vi "realTimeDisplay_AS3.vi"() -> ()   [LabVIEW 2016]
uses:
  <userlib>/RSA_API/RSA_API.lvlib
panel:
  in  "Cluster":T1 {"verticalUnit" items=["SpectrumVerticalUnit_dBm", "SpectrumVerticalUnit_Watt", "SpectrumVerticalUnit_Volt", "SpectrumVerticalUnit_Amp", "SpectrumVerticalUnit_dBmV"]; "window" items=["SpectrumWindow_Kaiser", "SpectrumWindow_Mil6dB", "SpectrumWindow_BlackmanHarris", "SpectrumWindow_Rectangle", "SpectrumWindow_FlatTop", "SpectrumWindow_Hann"]}
  out "settings out 2":T2 {"window" items=["SpectrumWindow_Kaiser", "SpectrumWindow_Mil6dB", "SpectrumWindow_BlackmanHarris", "SpectrumWindow_Rectangle", "SpectrumWindow_FlatTop", "SpectrumWindow_Hann"]; "verticalUnit" items=["SpectrumVerticalUnit_dBm", "SpectrumVerticalUnit_Watt", "SpectrumVerticalUnit_Volt", "SpectrumVerticalUnit_Amp", "SpectrumVerticalUnit_dBmV"]}
  in  "Done":bool
  in  "center freq":dbl
  in  "refLevel in":dbl
  in  "Trace number":u32(ring) items=["SpectrumTrace1", "SpectrumTrace2", "SpectrumTrace3"]
  out "traceData out":sgl[](graph)
  out "outTracePoints out":i32
  out "Trace Ready":bool
  out "enable out":bool
  out "refLevel out":dbl
  out "cf out":dbl
  in  "deviceID":i32
  out "deviceType out":string
  out "deviceSerial out":string
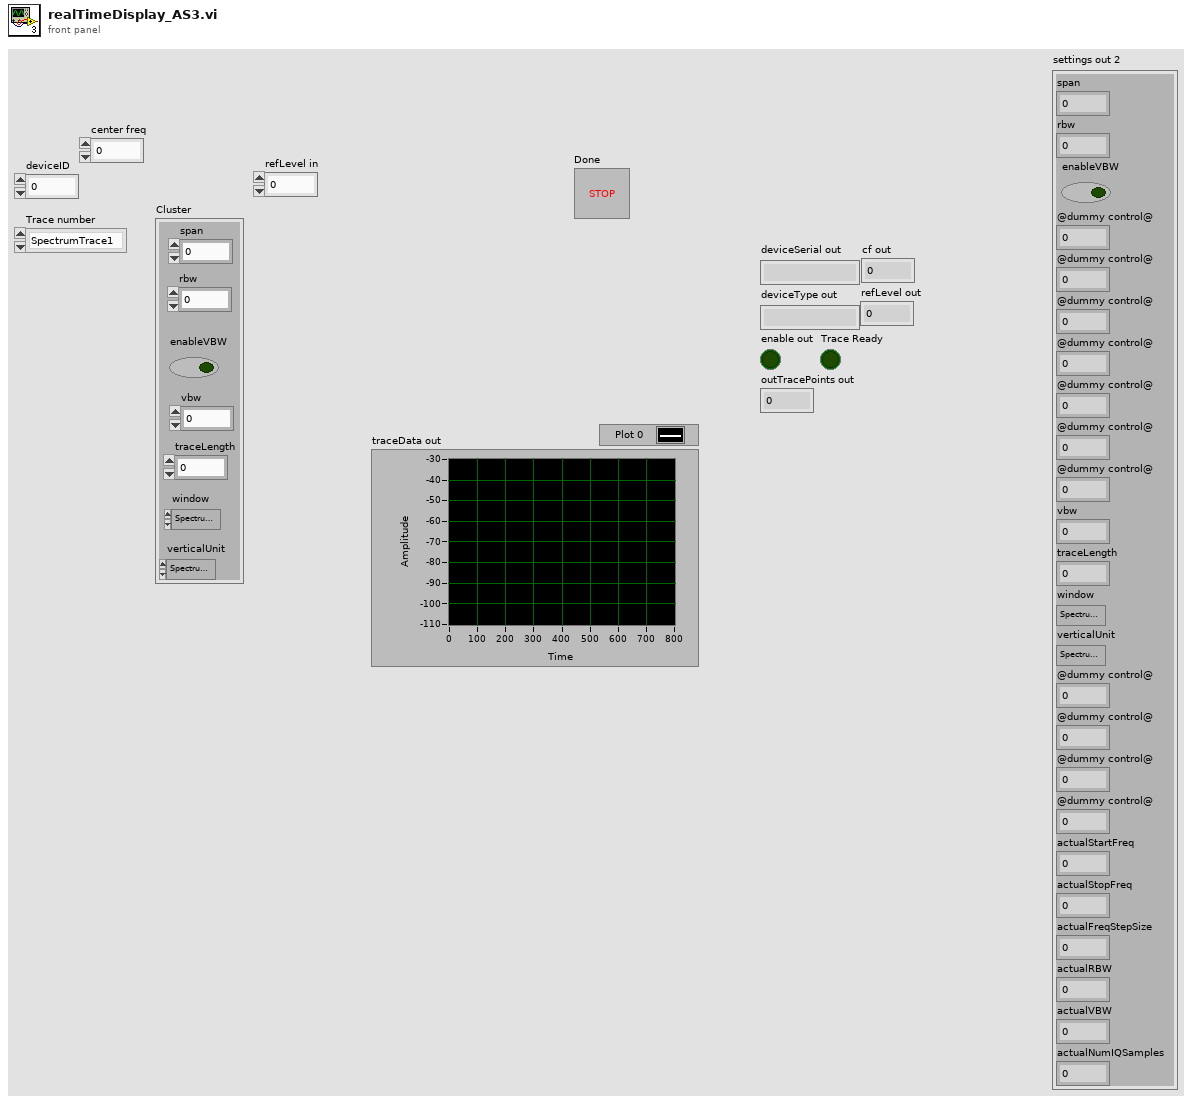
[diagram p1: front panel]
types:
  T1 = cluster{"span":dbl, "rbw":dbl, "enableVBW":bool, "vbw":dbl, "traceLength":i32, "window":u32, "verticalUnit":u32}
  T2 = cluster{"span":dbl, "rbw":dbl, "enableVBW":bool, "@dummy control@":i8, "@dummy control@":i8, "@dummy control@":i8, "@dummy control@":i8, "@dummy control@":i8, "@dummy control@":i8, "@dummy control@":i8, "vbw":dbl, "traceLength":i32, "window":u32, "verticalUnit":u32, "@dummy control@":i8, "@dummy control@":i8, "@dummy control@":i8, "@dummy control@":i8, "actualStartFreq":dbl, "actualStopFreq":dbl, "actualFreqStepSize":dbl, "actualRBW":dbl, "actualVBW":dbl, "actualNumIQSamples":i32}
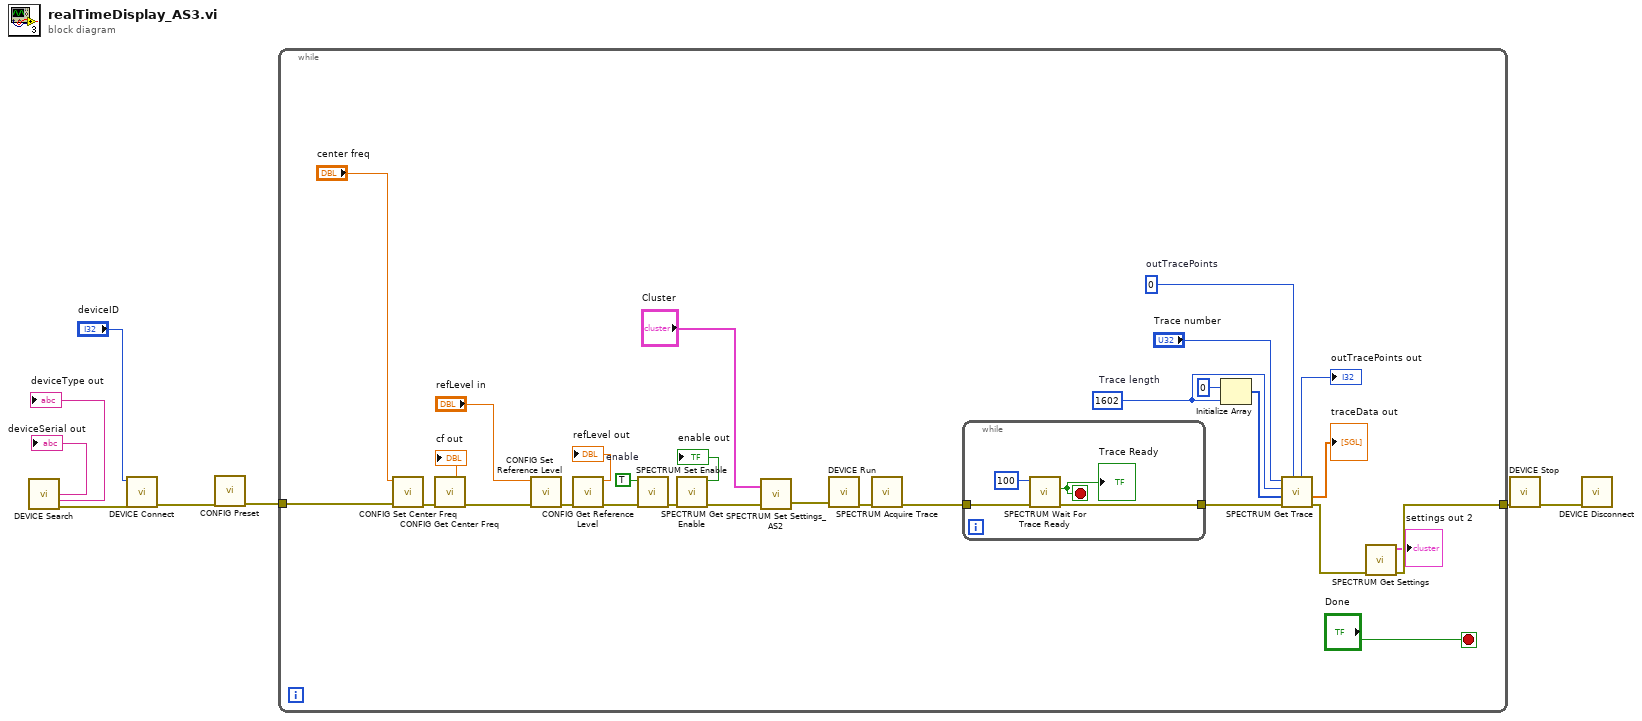
[diagram p0: block diagram]
diagram:
  n1 = call <userlib>:"DEVICE Search.vi"() -> ("deviceSerial out"=→"deviceSerial out":string, "deviceType out"=→"deviceType out":string, "error out"=w5:errorcluster)  [unwired: 10 in, 3 out]
  n2 = call <userlib>:"DEVICE Connect.vi"("error in (no error)"=w5, "deviceID"="deviceID") -> ("error out"=w4:errorcluster)  [unwired: 8 in, 1 out]
  n3 = call <userlib>:"CONFIG Preset.vi"("error in (no error)"=w4) -> ("error out"=w3:errorcluster)  [unwired: 9 in, 1 out]
  n4 = while {
    tunnel: w3 -> [w16]
    tunnel: [w13] -> w1
    stop <- "Done" stop-if-true
    w31 = TRUE  # enable
    w23 = 1602  # Trace length
    w24 = 0  # outTracePoints
    n5 = call <userlib>:"CONFIG Set Center Freq.vi"("error in (no error)"=w16, "cf"="center freq") -> ("error out"=w18:errorcluster)  [unwired: 8 in, 1 out]
    n6 = call <userlib>:"CONFIG Get Center Freq.vi"("error in (no error)"=w18) -> ("error out"=w37:errorcluster, "cf out"=→"cf out":dbl)  [unwired: 8 in, 1 out]
    n7 = call <userlib>:"CONFIG Set Reference Level.vi"("error in (no error)"=w37, "refLevel"="refLevel in") -> ("error out"=w36:errorcluster)  [unwired: 8 in, 1 out]
    n8 = call <userlib>:"CONFIG Get Reference Level.vi"("error in (no error)"=w36) -> ("error out"=w32:errorcluster, "refLevel out"=→"refLevel out":dbl)  [unwired: 8 in, 1 out]
    n9 = call <userlib>:"SPECTRUM Set Enable.vi"("error in (no error)"=w32, "enable"=w31) -> ("error out"=w30:errorcluster)  [unwired: 8 in, 1 out]
    n10 = call <userlib>:"SPECTRUM Get Enable.vi"("error in (no error)"=w30) -> ("error out"=w11:errorcluster, "enable out"=→"enable out":bool)  [unwired: 8 in, 1 out]
    n11 = call "SPECTRUM Set Settings_AS2.vi"("error in (no error)"=w11, "Cluster"="Cluster") -> ("error out"=w10:errorcluster)  [unwired: 1 out]
    n12 = call <userlib>:"DEVICE Run.vi"("error in (no error)"=w10) -> ("error out"=w28:errorcluster)  [unwired: 9 in, 1 out]
    n13 = call <userlib>:"SPECTRUM Acquire Trace.vi"("error in (no error)"=w28) -> ("error out"=w27:errorcluster)  [unwired: 9 in, 1 out]
    n14 = while {
      tunnel: w27 -> [w39]
      tunnel: [w38] -> w26
      stop <- w40 stop-if-true
      n15 = call <userlib>:"SPECTRUM Wait For Trace Ready.vi"("error in (no error)"=w39, "timeoutMsec"=100) -> ("error out"=w38:errorcluster, "ready out"=w40:bool)  [unwired: 7 in, 1 out]
      "Trace Ready" <- w40
    }
    n16 = Initialize Array(0 ("element"), w23) -> (w21:i32[])
    n17 = call <userlib>:"SPECTRUM Get Trace.vi"("outTracePoints"=w24, "error in (no error)"=w26, "traceData"=w21, "maxTracePoints"=w23, "trace"="Trace number") -> ("error out"=w14:errorcluster, "traceData out"=→"traceData out":sgl[], "outTracePoints out"=→"outTracePoints out":i32)  [unwired: 3 in, 1 out]
    n18 = call <userlib>:"SPECTRUM Get Settings.vi"("error in (no error)"=w14) -> ("error out"=w13:errorcluster, "settings out"=→"settings out 2":T2)  [unwired: 8 in, 1 out]
  }
  n19 = call <userlib>:"DEVICE Stop.vi"("error in (no error)"=w1) -> ("error out"=w2:errorcluster)  [unwired: 9 in, 1 out]
  n20 = call <userlib>:"DEVICE Disconnect.vi"("error in (no error)"=w2) -> ()  [unwired: 9 in, 2 out]
